vi "Save Class in SelfNode.vi"(8 "error in (no error)":errorcluster caption="错误输入（无错误）", 11 "PanelLinkNode 输入":refnum<class "PanelLinkNode.lvclass"> caption="DNL_LabVIEW Object in") -> (0 "error out":errorcluster caption="错误输出", 3 "PanelLinkNode 输出":refnum<class "PanelLinkNode.lvclass"> caption="DNL_LabVIEW Object out")   [LabVIEW 2013, in "PanelLinkNode.lvclass"]
uses:
  PanelLinkNode.lvclass
  PanelLinkNode.lvclass/PanelLinkNode.ctl
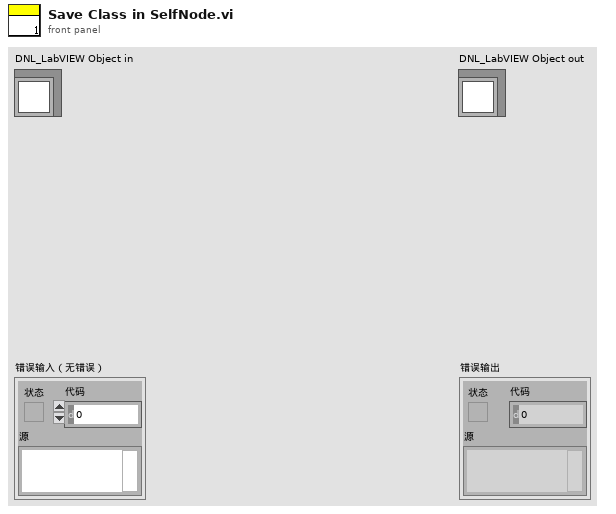
[diagram p1: front panel]
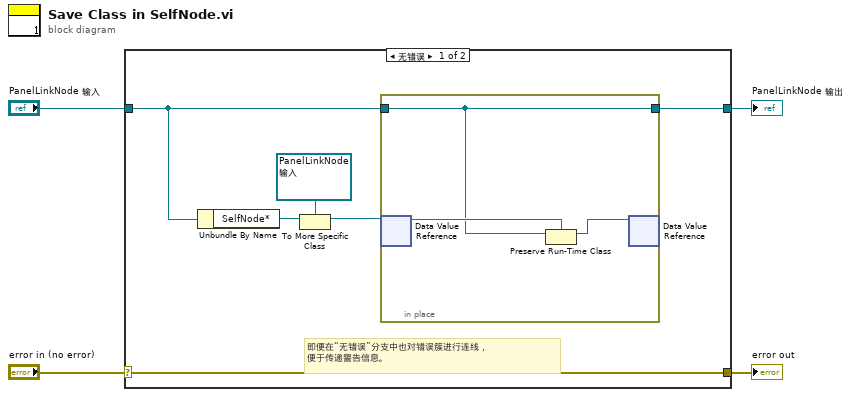
[diagram p0: block diagram]
diagram:
  n1 = case shown="无错误" "error in (no error)" {
    selector: "error in (no error)" -> [w10 w15]
    tunnel: [w10 w15] -> w3
    tunnel: [w5 w14] -> w1
    tunnel: "PanelLinkNode 输入" -> [w6 w14]
    frame No Error {
      # "即便在“无错误”分支中也对错误簇进行连线，\n便于传递警告信息。"
      n2 = Unbundle By Name(w6) -> ("SelfNode*"=w9:refnum<data-value>)
      n3 = To More Specific Class(target class=refnum<data-value> refnum ("数据值引用"), reference=w9) -> (specific class reference=w7:refnum<data-value>)  [unwired: 1 in, 1 out]
      n4 = in-place {
        in-place-border: w6 -> [w11]
        in-place-border: [w11] -> w5
        n5 = in-place-dvr #1(w7) -> (w13:refnum<class "PanelLinkNode.lvclass">)  [unwired: 1 out]
        n6 = Preserve Run-Time Class(object in=w11, 2:w13) -> (object out=w12:refnum<class "PanelLinkNode.lvclass">)  [unwired: 1 in, 1 out]
        n7 = in-place-dvr #1(w12) -> ()  [unwired: 2 out]
      }
    }
    frame Error {
    }
  }
  "error out" <- w3
  "PanelLinkNode 输出" <- w1
